vi "MFC.vi"(7 "delay (ms)":u32=500, 8 "error in (no error)":errorcluster caption="에러 입력(에러 없음)", 10 "열거형":enum16{"1", "2", "3"}(ring), 11 "Port":refnum<visa-resource-name>="COM1") -> (0 "error out":errorcluster, 3 "flow":sgl format="%.3g")   [LabVIEW 2015]
uses:
  MFC_Address.ctl
  Program Files (x86)/National Instruments/LabVIEW 2015/examples/Instrument IO/Serial/support/Serial - Settings.ctl
  <vilib>/Instr/_visa.llb/VISA Configure Serial Port (Instr).vi
panel:
  out "Response":T1
  out "bytes read 2":u32
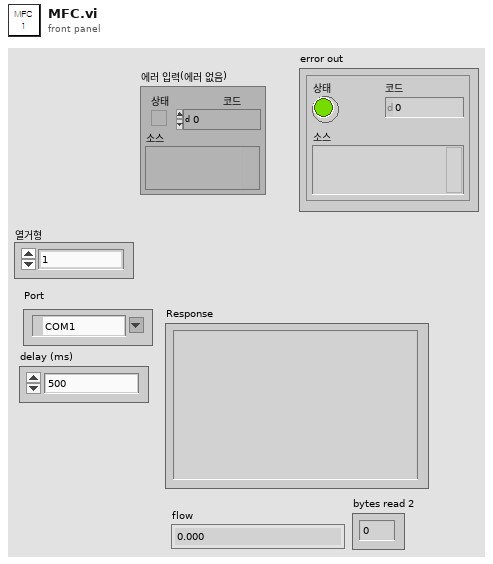
[diagram p1: front panel]
types:
  T1 = typedef "MFC_Address.ctl" = string
  T2 = typedef "Serial - Settings.ctl" = cluster{"baud rate":u32, "data bits":u16, "parity":enum16{"None", "Odd", "Even", "Mark", "Space"}, "stop bits":u16, "flow control":u16}
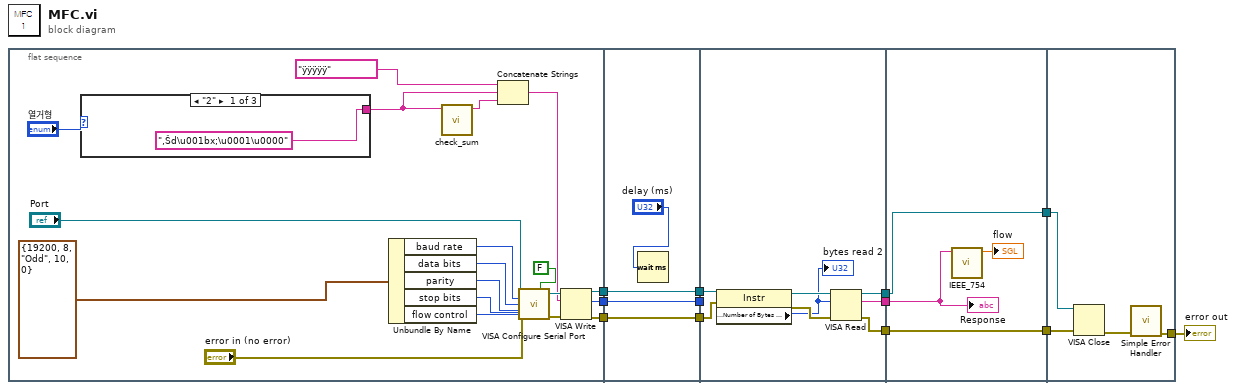
[diagram p0: block diagram]
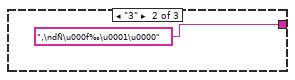
[diagram p2: hidden frame]
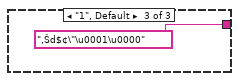
[diagram p3: hidden frame]
diagram:
  n1 = flat-sequence {
    tunnel: [w20] -> w12
    tunnel: [w19] -> w11
    tunnel: [w18] -> w10
    tunnel: w12 -> [w37]
    tunnel: w11 -> [w35]
    tunnel: w10 -> [w38]
    tunnel: [w38] -> w9
    tunnel: [w37] -> w8
    tunnel: [w35] -> w7
    tunnel: w9 -> [_]
    tunnel: w8 -> [w43]
    tunnel: [w42] -> w6
    tunnel: [w41] -> w5
    tunnel: w7 -> [w40]
    tunnel: [w39] -> w4
    tunnel: w6 -> [w49]
    tunnel: [w50] -> w3
    tunnel: w5 -> [w50]
    tunnel: [w47] -> w2
    tunnel: w4 -> [w47]
    tunnel: w3 -> [w53]
    tunnel: [w52] -> w1
    tunnel: w2 -> [w51]
    frame #0 {
      n2 = case shown="\"2\"" "열거형" {
        tunnel: ["‚Šd\u001bx;\u0001\u0000" ("Command") "‚\ndÑ\u000f‰\u0001\u0000" ("Command") "‚Šd$¢\"\u0001\u0000" ("Command")] -> w15
        frame "2" {
        }
        frame "3" {
        }
        frame "1", Default {
        }
      }
      n3 = Unbundle By Name(T2 {"baud rate"=19200, "data bits"=8, "parity"=enum."Odd", "stop bits"=10, "flow control"=0} ("Serial Settings")) -> ("baud rate"=w25:u32, "data bits"=w24:u16, "parity"=w23:enum16{"None", "Odd", "Even", "Mark", "Space"}, "stop bits"=w22:u16, "flow control"=w21:u16)
      n4 = call "check_sum.vi"("command"=w15) -> ("Check Sum"=w17:string)  [unwired: 10 in]
      n5 = Concatenate Strings("ÿÿÿÿÿ" ("문자열"), w15, w17) -> (w27:string)
      n6 = call-poly "VISA Configure Serial Port"("VISA resource name"="Port", "Enable Termination\nChar (T)"=FALSE ("종료문자활성화"), "baud rate (9600)"=w25, "data bits (8)"=w24, "parity (0:none)"=w23, "error in (no error)"="error in (no error)", "stop bits (10: 1 bit)"=w22, "flow control (0:none)"=w21) -> ("VISA resource name out"=w29:refnum<visa-resource-name>, "error out"=w30:errorcluster)  [unwired: 1 in, 5 out]
      n7 = VISA Write(VISA resource name=w29, write buffer=w27, error in (no error)=w30) -> (VISA resource name out=w20:refnum<visa-resource-name>, return count=w18:u32, error out=w19:errorcluster)
    }
    frame #1 {
      n8 = Wait (ms)(milliseconds to wait="delay (ms)") -> ()  [unwired: 1 out]
    }
    frame #2 {
      n9 = property class="Instr"(reference=w43, error in=w40) -> (reference out=w46:refnum<visa-resource-name>, error out=w45:errorcluster, "Serial Settings:Number of Bytes at Serial Port"=w44:u32)
      "bytes read 2" <- w44
      n10 = VISA Read(VISA resource name=w46, byte count=w44, error in (no error)=w45) -> (VISA resource name out=w41:refnum<visa-resource-name>, read buffer=w42:string, error out=w39:errorcluster)  [unwired: 1 out]
    }
    frame #3 {
      n11 = call "IEEE_754.vi"("input"=w49) -> ("Return"=→"flow":sgl)  [unwired: 10 in]
      "Response" <- w49
    }
    frame #4 {
      n12 = VISA Close(VISA resource name=w53, error in (no error)=w51) -> (error out=w54:errorcluster)
      n13 = call <vilib>:"Simple Error Handler.vi"("error in (no error)"=w54) -> ("error out"=w52:errorcluster)  [unwired: 1 in, 7 out]
    }
  }
  "error out" <- w1
